vi "nominal ingest avro stream.vi"(7 "out_job":i32, 8 "error in (no error)":errorcluster, 9 "dataset_rid":string, 10 "file_path":string, 11 "client":i32) -> (0 "error out":errorcluster, 3 "function return":i32, 5 "out_job out":i32)   [LabVIEW 2020, in "client.lvlib"]
doc: "int32_t nominal_ingest_avro_stream(int32_t client,\n const char *file_path,\n const char *dataset_rid,\n int32_t *out_job);"
uses:
  client.lvlib
  bin/nominalClient_64.dll
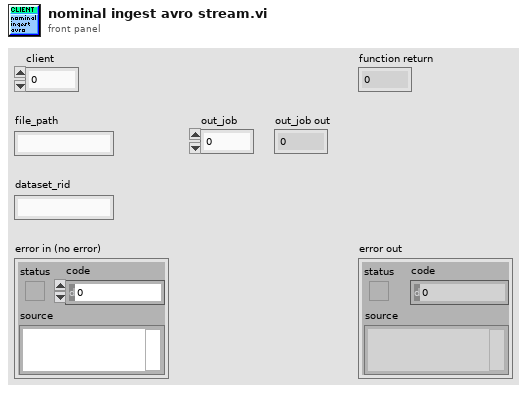
[diagram p1: front panel]
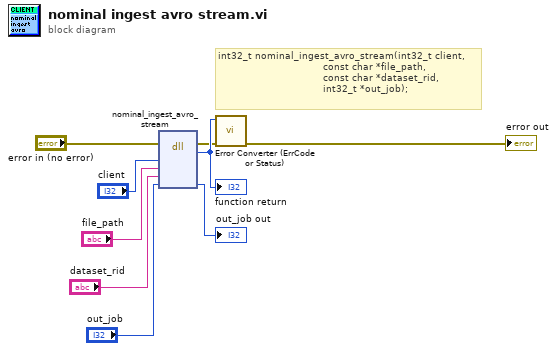
[diagram p0: block diagram]
diagram:
  # "int32_t nominal_ingest_avro_stream(int32_t client,\n                                   const char *file_path,\n                                   const char *dataset_rid,\n                                   int32_t *out_job);"
  n1 = dll-call lib="C:/code/labview-client-rs/lv_src/bin/nominalClient_*.*" fn="nominal_ingest_avro_stream"(error in="error in (no error)", "client"="client", "file_path"="file_path", "dataset_rid"="dataset_rid", "out_job"="out_job") -> (error out=w2:errorcluster, w9:i32, "out_job"=→"out_job out":i32)  [unwired: 5 in, 1 out]
  "function return" <- w9
  n2 = call "Error Converter (ErrCode or Status).vi"("error in (no error)"=w2, "error code"=w9) -> ("error out"=→"error out":errorcluster)  [unwired: 9 in]
